vi "Benchmarking Maps.vi"() -> ()   [LabVIEW 2019]
uses:
  <vilib>/Utility/miscctls.llb/LVMapReplaceAction.ctl
  60997348-983d-410f-b173-2636c18fe73e.vi
  <vilib>/Analysis/baseanly.llb/Mean (DBL).vi
  <vilib>/Analysis/NI_AALBase.lvlib
panel:
  out "Find table items":cluster{"Entry Count":i32[], dbl[]}[](graph)
  out "Build table data":cluster{"Entry Count":i32[], dbl[]}[](graph)
  out "Time to find array items":dbl
  out "Time to find IPE items":dbl
  out "Time to look in map":dbl
  out "Time to build map table":dbl
  out "Variant Attributes":string[](array[string])
  out "Array":string[](array[string])
  out "IPE":string[](array[string])
  out "Look in Map":string[](array[string])
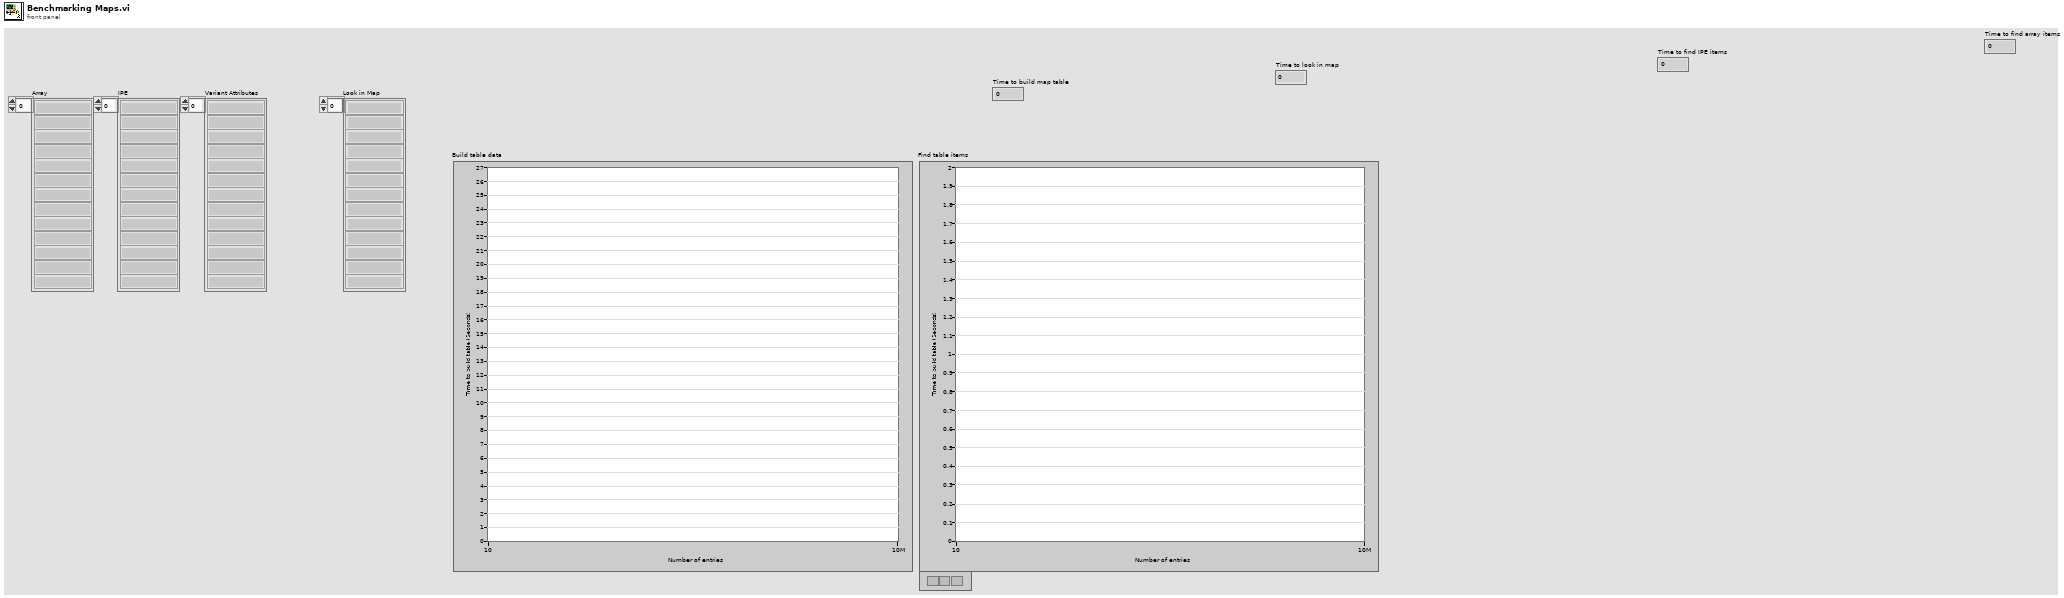
[diagram p1: front panel]
types:
  T1 = typedef "LVMapReplaceAction.ctl" = enum32{"Modify Entry only if found", "Add or Modify Entry", "Delete Entry"}
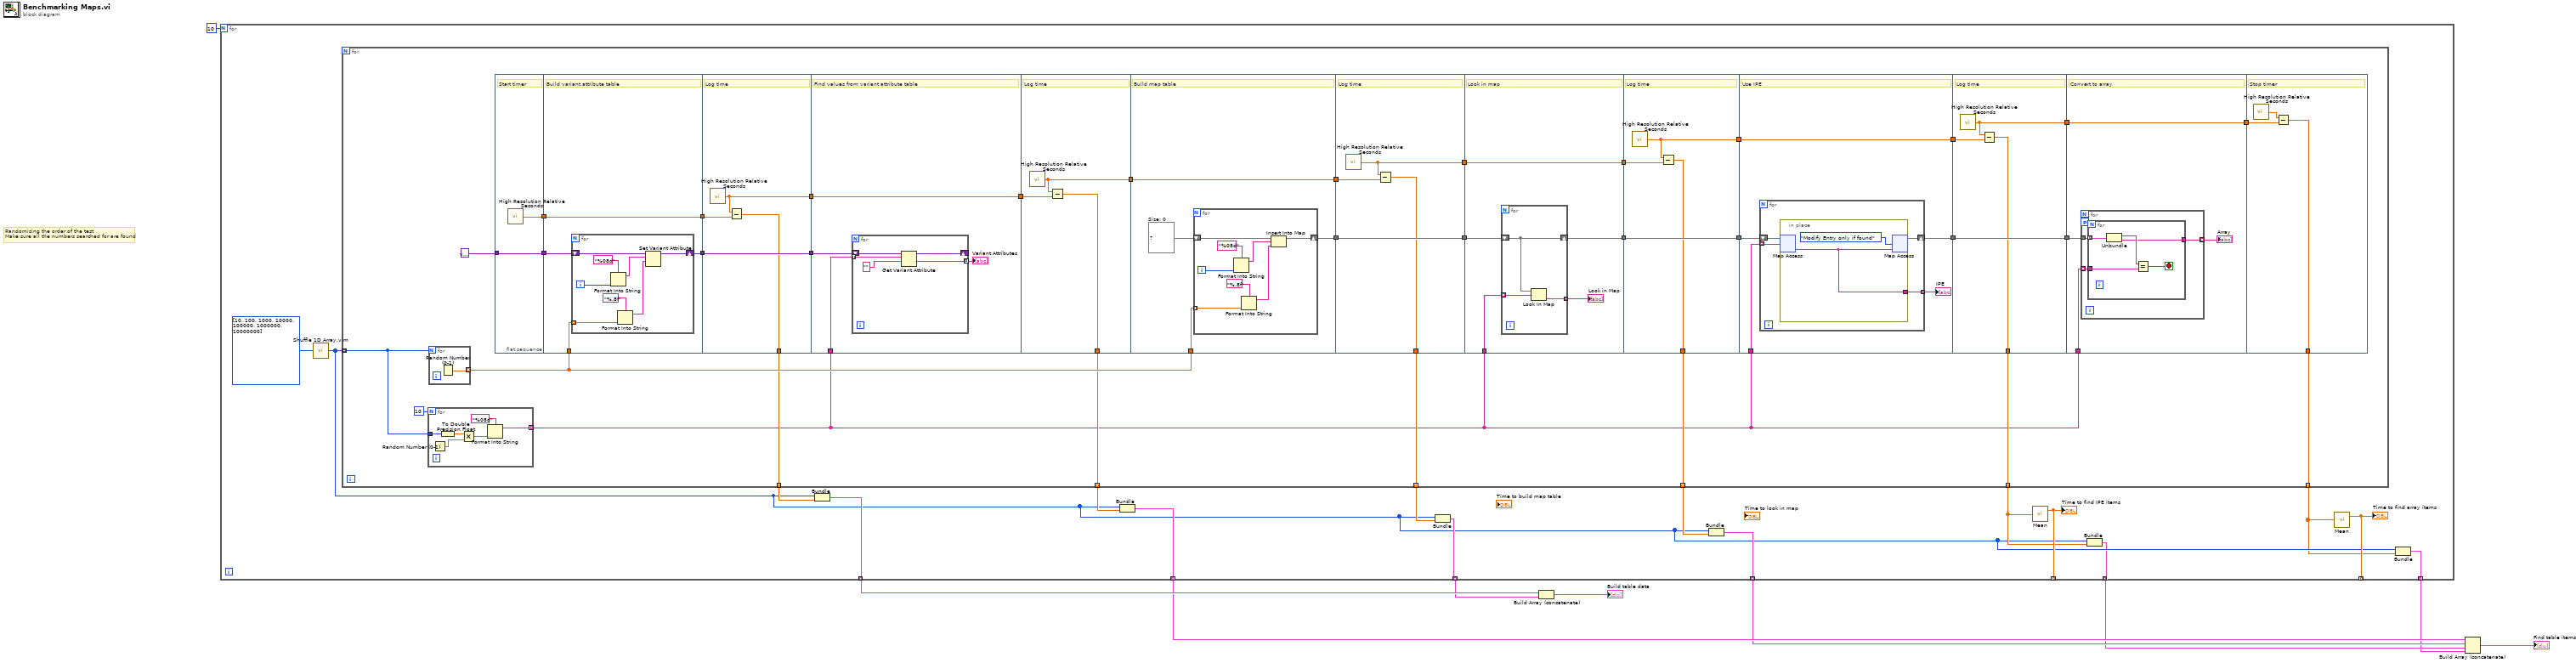
[diagram p0: block diagram]
diagram:
  # "Randomising the order of the test\nMake sure all the numbers searched for are found"
  n1 = for {
    N: 10 -> [_]
    tunnel: [w25] -> _ mode=indexing
    tunnel: [w24] -> _ mode=indexing
    tunnel: [w20] -> w8 mode=indexing
    tunnel: [w19] -> w5 mode=indexing
    tunnel: [w17] -> w7 mode=indexing
    tunnel: [w15] -> w4 mode=indexing
    tunnel: [w11] -> w3 mode=indexing
    tunnel: [w10] -> w2 mode=indexing
    n2 = call "Shuffle 1D Array.vim"("array"=i32[] [10, 100, 1000, 10000, 100000, 1000000, 10000000] ("Entry Count")) -> ("shuffled array"=w13:i32[])  [unwired: 4 in]
    n3 = for {
      tunnel: [w34] -> w22 mode=indexing
      tunnel: [w33] -> w21 mode=indexing
      tunnel: [w32] -> w18 mode=indexing
      tunnel: [w31] -> w16 mode=indexing
      tunnel: [w30] -> w14 mode=indexing
      tunnel: [w29] -> w12 mode=indexing
      tunnel: w13 -> [w27] mode=indexing
      n4 = for {
        N: 10 -> [_]
        tunnel: w27 -> [w62]
        tunnel: [w58] -> w26 mode=indexing
        n5 = Random Number (0-1)() -> (number: 0 to 1=w63:dbl)
        n6 = To Double Precision Float(number=w62) -> (double precision float=w61:dbl)
        n7 = Multiply(x=w61, y=w63) -> (x*y=w60:dbl)
        n8 = Format Into String(format string="%08d", w60) -> (resulting string=w58:string)  [unwired: 2 in, 1 out]
      }
      n9 = for {
        N: w27 -> [_]
        tunnel: [w152] -> w35 mode=indexing
        n10 = Random Number (0-1)() -> (number: 0 to 1=w152:dbl)
      }
      n11 = flat-sequence {
        tunnel: variant -> [w65]
        tunnel: [w65] -> w57
        tunnel: [w64] -> w56
        tunnel: [w68] -> w55
        tunnel: w57 -> [w69]
        tunnel: w35 -> [w67]
        tunnel: w56 -> [w66]
        tunnel: [w66] -> w54
        tunnel: w55 -> [w81]
        tunnel: [w81] -> w53
        tunnel: w54 -> [w80]
        tunnel: [w79] -> w52
        tunnel: [w78] -> w34
        tunnel: w53 -> [w84]
        tunnel: w26 -> [w83]
        tunnel: w52 -> [w82]
        tunnel: [w82] -> w51
        tunnel: w51 -> [w93]
        tunnel: [w92] -> w50
        tunnel: [w91] -> w33
        tunnel: w35 -> [w96]
        tunnel: [w95] -> w49
        tunnel: w50 -> [w94]
        tunnel: [w94] -> w48
        tunnel: [w109] -> w47
        tunnel: w49 -> [w109]
        tunnel: w48 -> [w108]
        tunnel: [w107] -> w46
        tunnel: [w106] -> w32
        tunnel: w26 -> [w113]
        tunnel: w47 -> [w112]
        tunnel: [w111] -> w45
        tunnel: w46 -> [w110]
        tunnel: [w110] -> w44
        tunnel: [w121] -> w43
        tunnel: w45 -> [w121]
        tunnel: w44 -> [w120]
        tunnel: [w119] -> w42
        tunnel: [w118] -> w31
        tunnel: w26 -> [w125]
        tunnel: w43 -> [w123]
        tunnel: [w124] -> w41
        tunnel: w42 -> [w122]
        tunnel: [w122] -> w40
        tunnel: w41 -> [w136]
        tunnel: [w136] -> w39
        tunnel: w40 -> [w135]
        tunnel: [w134] -> w38
        tunnel: [w133] -> w30
        tunnel: w39 -> [w139]
        tunnel: w26 -> [w138]
        tunnel: [w137] -> w37
        tunnel: w38 -> [w137]
        tunnel: w37 -> [w151]
        tunnel: [w149] -> w29
        frame #0 {
          # "Start timer"
          n12 = call <vilib>:"High Resolution Relative Seconds.vi"() -> ("relative seconds"=w64:dbl)
        }
        frame #1 {
          # "Build variant attribute table"
          n13 = for {
            shift-right: [w76] -> w68
            shift-left: w69 -> [w77]
            tunnel: w67 -> [w70] mode=indexing
            i -> [w73]
            n14 = Format Into String(format string="%08d", w73) -> (resulting string=w72:string)  [unwired: 2 in, 1 out]
            n15 = Format Into String(format string="%.8f", w70) -> (resulting string=w71:string)  [unwired: 2 in, 1 out]
            n16 = Set Variant Attribute(Variant=w77, name=w72, value=w71) -> (Variant out=w76:variant)  [unwired: 1 in, 2 out]
          }
        }
        frame #2 {
          # "Log time"
          n17 = call <vilib>:"High Resolution Relative Seconds.vi"() -> ("relative seconds"=w79:dbl)
          n18 = Subtract(x=w79, y=w80) -> (x-y=w78:dbl)
        }
        frame #3 {
          # "Find values from variant attribute table"
          n19 = for {
            shift-right: [w89] -> _
            shift-left: w84 -> [w90]
            tunnel: w83 -> [w88] mode=indexing
            tunnel: [w86] -> w85 mode=indexing
            n20 = Get Variant Attribute(Variant=w90, name=w88, default value (empty Variant)="") -> (duplicate Variant=w89:variant, value=w86:string)  [unwired: 1 in, 2 out]
          }
          "Variant Attributes" <- w85
        }
        frame #4 {
          # "Log time"
          n21 = call <vilib>:"High Resolution Relative Seconds.vi"() -> ("relative seconds"=w92:dbl)
          n22 = Subtract(x=w92, y=w93) -> (x-y=w91:dbl)
        }
        frame #5 {
          w97 = map{string, string} {}  # Size: 0
          # "Build map table"
          n23 = for {
            shift-right: [w104] -> w95
            shift-left: w97 -> [w105]
            tunnel: w96 -> [w98] mode=indexing
            i -> [w102]
            n24 = Format Into String(format string="%08d", w102) -> (resulting string=w103:string)  [unwired: 2 in, 1 out]
            n25 = Format Into String(format string="%.8f", w98) -> (resulting string=w100:string)  [unwired: 2 in, 1 out]
            n26 = Insert Into Map(map in=w105, key=w103, value=w100) -> (map out=w104:map{string, string})  [unwired: 2 out]
          }
        }
        frame #6 {
          # "Log time"
          n27 = call <vilib>:"High Resolution Relative Seconds.vi"() -> ("relative seconds"=w107:dbl)
          n28 = Subtract(x=w107, y=w108) -> (x-y=w106:dbl)
        }
        frame #7 {
          # "Look in map"
          n29 = for {
            tunnel: w113 -> [w117] mode=indexing
            shift-right: [w116] -> w111
            shift-left: w112 -> [w116]
            tunnel: [w115] -> w114 mode=indexing
            n30 = Look In Map(map=w116, key=w117) -> (value=w115:string)  [unwired: 1 in, 1 out]
          }
          "Look in Map" <- w114
        }
        frame #8 {
          # "Log time"
          n31 = call <vilib>:"High Resolution Relative Seconds.vi"() -> ("relative seconds"=w119:dbl)
          n32 = Subtract(x=w119, y=w120) -> (x-y=w118:dbl)
        }
        frame #9 {
          # "Use IPE"
          n33 = for {
            shift-right: [w129] -> w124
            shift-left: w123 -> [w130]
            tunnel: w125 -> [w128] mode=indexing
            tunnel: [w127] -> w126 mode=indexing
            n34 = in-place {
              in-place-border: [w131] -> w127
              n35 = in-place-map #1(w130, w128) -> (w131:string)  [unwired: 1 in, 1 out]
              n36 = in-place-map #1(w131, LVMapReplaceAction."Modify Entry only if found" ("action")) -> (w129:map{string, string})  [unwired: 2 out]
            }
          }
          "IPE" <- w126
        }
        frame #10 {
          # "Log time"
          n37 = call <vilib>:"High Resolution Relative Seconds.vi"() -> ("relative seconds"=w134:dbl)
          n38 = Subtract(x=w134, y=w135) -> (x-y=w133:dbl)
        }
        frame #11 {
          # "Convert to array"
          n39 = for {
            tunnel: w139 -> [w143]
            tunnel: w138 -> [w142] mode=indexing
            tunnel: [w141] -> w140 mode=indexing
            workers-P: _ -> [_]
            n40 = for {
              tunnel: w143 -> [w148] mode=indexing
              tunnel: w142 -> [w146]
              tunnel: [w145] -> w141
              stop <- w144 stop-if-true
              n41 = Unbundle(w148) -> (w147:string, w145:string)
              n42 = Equal?(x=w147, y=w146) -> (x = y?=w144:bool)
            }
          }
          "Array" <- w140
        }
        frame #12 {
          # "Stop timer"
          n43 = call <vilib>:"High Resolution Relative Seconds.vi"() -> ("relative seconds"=w150:dbl)
          n44 = Subtract(x=w150, y=w151) -> (x-y=w149:dbl)
        }
      }
    }
    n45 = Bundle("shuffled array"=w13, w22) -> (w20:cluster{"shuffled array":i32[], dbl[]})  [unwired: 1 in]
    n46 = Bundle("shuffled array"=w13, w21) -> (w19:cluster{"shuffled array":i32[], dbl[]})  [unwired: 1 in]
    n47 = Bundle("shuffled array"=w13, w18) -> (w17:cluster{"shuffled array":i32[], dbl[]})  [unwired: 1 in]
    n48 = Bundle("shuffled array"=w13, w16) -> (w15:cluster{"shuffled array":i32[], dbl[]})  [unwired: 1 in]
    n49 = call-poly <vilib>:"Mean.vi"("X"=w14) -> ("mean"=w25:dbl)  [unwired: 1 out]
    "Time to find IPE items" <- w25
    n50 = Bundle("shuffled array"=w13, w14) -> (w11:cluster{"shuffled array":i32[], dbl[]})  [unwired: 1 in]
    n51 = call-poly <vilib>:"Mean.vi"("X"=w12) -> ("mean"=w24:dbl)  [unwired: 1 out]
    "Time to find array items" <- w24
    n52 = Bundle("shuffled array"=w13, w12) -> (w10:cluster{"shuffled array":i32[], dbl[]})  [unwired: 1 in]
  }
  n53 = Build Array (concatenate)(w8, w7) -> (→"Build table data":cluster{"shuffled array":i32[], dbl[]}[])
  n54 = Build Array (concatenate)(w5, w4, w3, w2) -> (→"Find table items":cluster{"shuffled array":i32[], dbl[]}[])
